vi "From Unix Time.vi"(0 "unix time":u32) -> (2 "timestamp":timestamp)   [LabVIEW 2013, in "libssh2.lvlib"]
doc: "Convert UNIX time to LabVIEW time."
uses:
  libssh2.lvlib
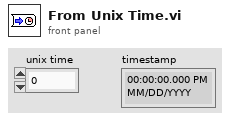
[diagram p1: front panel]
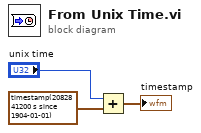
[diagram p0: block diagram]
diagram:
  n1 = Add(x="unix time", y=timestamp(2082841200 s since 1904-01-01)) -> (x+y=→"timestamp":timestamp)
